vi "Set LogicIO by Label.vi"(8 "error in (no error)":errorcluster, 10 "LogicIO obj":refnum<class "LogicIO.lvclass">, 11 "VacuumLine in":refnum<class "VacuumLine.lvclass">) -> (0 "error out":errorcluster, 3 "VacuumLine out":refnum<class "VacuumLine.lvclass">)   [LabVIEW 2016, in "Hardware.lvlib" / "VacuumLine.lvlib" / "VacuumLine.lvclass"]
uses:
  <userlib>/Common Components/Hardware/Abstract System/VacuumLine/VacuumLine/VacuumLine.lvclass
  <userlib>/Common Components/Hardware/LogicIO/LogicIO/LogicIO.lvclass
  C:/Program Files (x86)/National Instruments/LabVIEW 2016/user.lib/Common Components/Hardware/Abstract Hardware/Hardware.lvclass
  <userlib>/Common Components/Hardware/Abstract System/VacuumLine/VacuumLine/VacuumLine.lvclass/VacuumLine.ctl
  <userlib>/Common Components/Hardware/Abstract Hardware/Hardware.lvclass/Hardware.ctl
  <userlib>/Common Components/Hardware/Abstract Hardware/Read Label.vi
panel:
  # "Reconnect on error!\nAssume already initialized if no error."
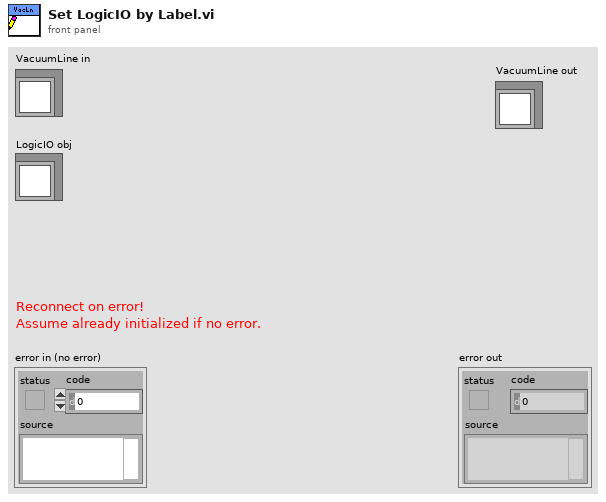
[diagram p1: front panel]
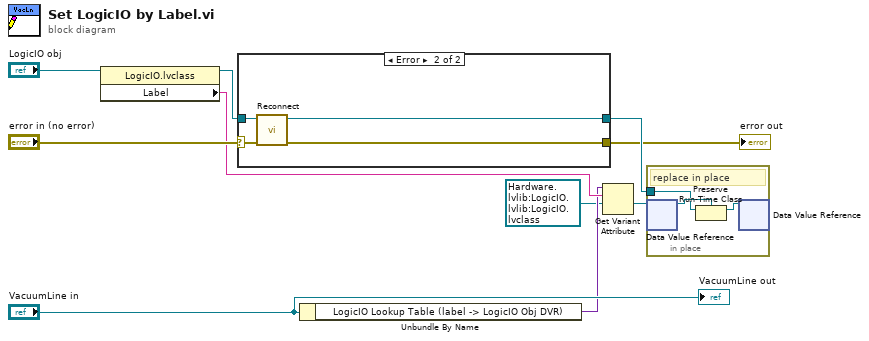
[diagram p0: block diagram]
diagram:
  n1 = property class="LogicIO.lvclass"(reference="LogicIO obj") -> (reference out=w9:refnum<class "LogicIO.lvclass">, "Label"=w6:string)  [unwired: 1 in, 1 out]
  n2 = case shown="Error" "error in (no error)" {
    selector: "error in (no error)" -> [w12 w13]
    tunnel: w9 -> [w11 w16]
    tunnel: [w11 w15] -> w2
    tunnel: [w12 w14] -> w1
    frame No Error {
    }
    frame Error {
      n3 = call-dynamic "Reconnect.vi"("error in (With error)"=w13, "Hardware in"=w16) -> ("error out"=w14:errorcluster, "Hardware out"=w15:refnum<class "LogicIO.lvclass">)  [unwired: 7 in, 1 out]
    }
  }
  "error out" <- w1
  n4 = Unbundle By Name("VacuumLine in") -> ("LogicIO Lookup Table (label -> LogicIO Obj DVR)"=w5:variant)
  n5 = Get Variant Attribute(Variant=w5, name=w6, default value (empty Variant)=refnum<data-value> refnum ("data value reference")) -> (value=w3:refnum<data-value>)  [unwired: 1 in, 3 out]
  n6 = in-place {
    in-place-border: w2 -> [w18]
    # "replace in place"
    n7 = in-place-dvr #1(w3) -> (w19:refnum<class "LogicIO.lvclass">)  [unwired: 1 out]
    n8 = Preserve Run-Time Class(object in=w18, 2:w19) -> (object out=w17:refnum<class "LogicIO.lvclass">)  [unwired: 1 in, 1 out]
    n9 = in-place-dvr #1(w17) -> ()  [unwired: 2 out]
  }
  "VacuumLine out" <- "VacuumLine in"
